vi "Update Explorer Tree.vi"(8 "error in (no error)":errorcluster, 10 "Explorer Tree":refnum<vi>, 11 "Project in":refnum<class "Project.lvclass">) -> (0 "error out":errorcluster, 3 "Project out":refnum<class "Project.lvclass">)   [LabVIEW 2015, in "Editor.lvclass"]
uses:
  Editor.lvclass
  Project.lvclass
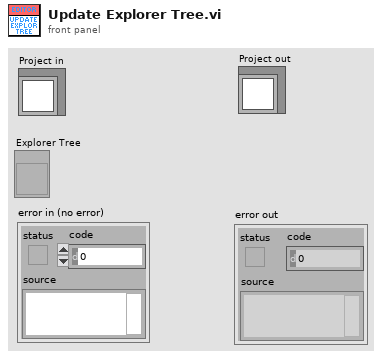
[diagram p1: front panel]
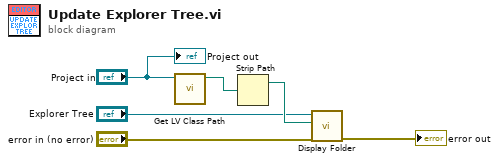
[diagram p0: block diagram]
diagram:
  n1 = call <vilib>:"Get LV Class Path.vi"("object"="Project in") -> ("class path"=w6:path)  [unwired: 9 in, 1 out]
  n2 = Strip Path(path=w6) -> (stripped path=w5:path)  [unwired: 1 out]
  n3 = call "Display Folder.vi"("error in (no error)"="error in (no error)", "Folder in"=w5, "TreeControl in"="Explorer Tree") -> ("error out"=→"error out":errorcluster)  [unwired: 6 in, 2 out]
  "Project out" <- "Project in"
